vi "Send Software Trigger.vi"(8 "error in (no error)":errorcluster, 11 "VISA resource name":refnum<visa-resource-name>) -> (0 "error out":errorcluster, 3 "VISA resource name out":refnum<visa-resource-name>)   [LabVIEW 2026, in "Agilent 33XXX Series.lvlib"]
doc: "Sends a software bus trigger to the instrument. You can use software bus triggers to trigger a frequency sweep. You must first set Trigger Source in the <B>Configure Trigger VI</B> to Software. \n\nNote:\nThis VI does not check the instrument status. If you want to check the instrument status, call the <B>Error Query VI</B> at the conclusion of your sweep operation."
uses:
  Agilent 33XXX Series.lvlib
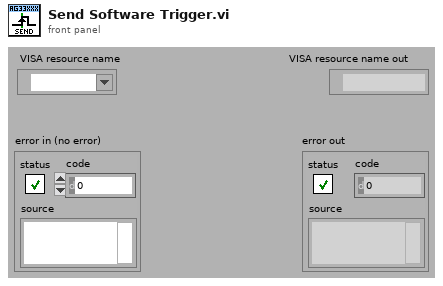
[diagram p1: front panel]
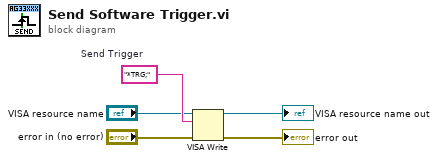
[diagram p0: block diagram]
diagram:
  w5 = "*TRG;"  # Send Trigger
  n1 = VISA Write(VISA resource name="VISA resource name", write buffer=w5, error in (no error)="error in (no error)") -> (VISA resource name out=→"VISA resource name out":refnum<visa-resource-name>, error out=→"error out":errorcluster)  [unwired: 1 out]
